vi "Build_Asylum_GetDevices.vi"(8 "error in (no error)":errorcluster, 11 "textWave":string="textWave") -> (0 "error out":errorcluster, 3 "Command":string)   [LabVIEW 2019]
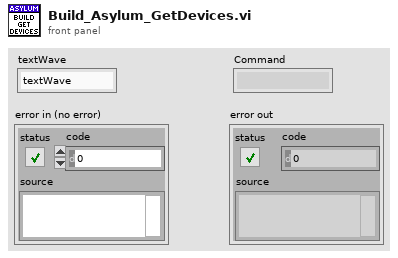
[diagram p1: front panel]
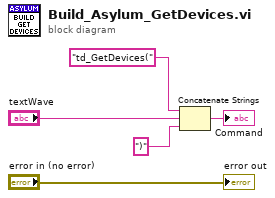
[diagram p0: block diagram]
diagram:
  n1 = Concatenate Strings("td_GetDevices(", "textWave", ")" ("string")) -> (→"Command":string)
  "error out" <- "error in (no error)"
